vi "Basic_smooth.vi"(0 "Smoothing":enum16{"Linear", "Logarithmic"}(ring), 2 "X array in":dbl[](array[numeric]) format="%.2f", 3 "Y array in":dbl[](array[numeric]) format="%.2f", 4 "No of estimates output":i32=1) -> (5 "X array Out":dbl[](array[numeric]) format="%.2f", 6 "Y array Out":dbl[](array[numeric]) format="%.2f")   [LabVIEW 2010]
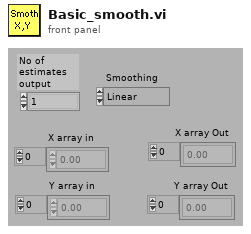
[diagram p1: front panel]
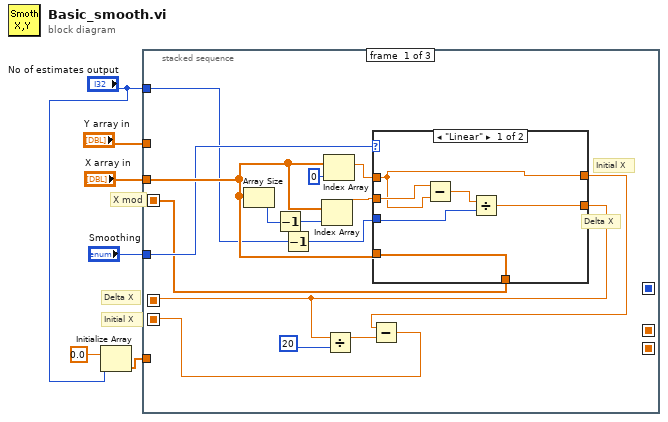
[diagram p0: block diagram]
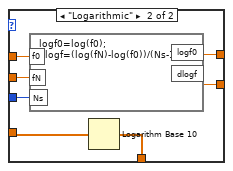
[diagram p2: hidden frame]
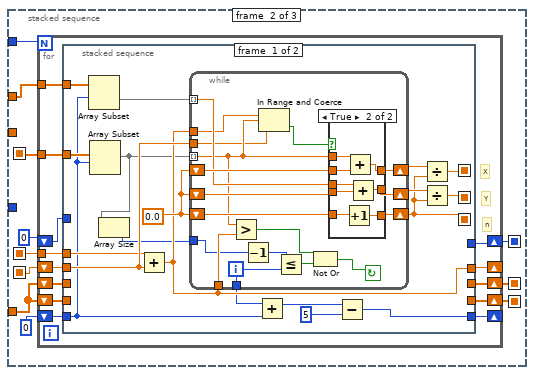
[diagram p3: hidden frame]
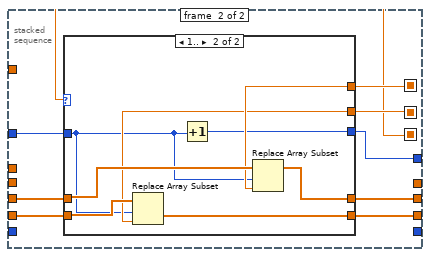
[diagram p5: hidden frame]
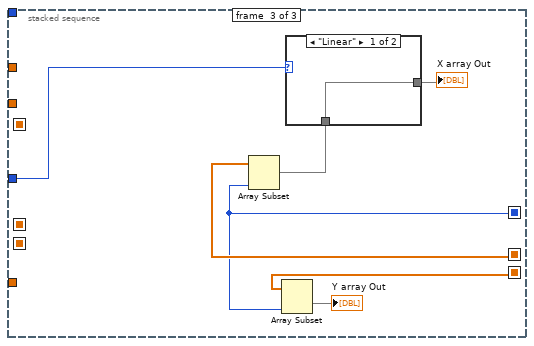
[diagram p7: hidden frame]
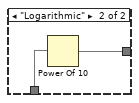
[diagram p8: hidden frame]
diagram:
  # "Initial X"
  # "Delta X"
  # "X mod"
  n1 = Initialize Array(0.0, "No of estimates output") -> (w2:dbl[])
  n2 = stacked-sequence {
    seq-local: [w11 _ _] -> [_ w43 _]
    seq-local: [w7 _ _] -> [_ w42 _]
    seq-local: [w14 _ _] -> [_ w44 _]
    seq-local: [_ w39 _] -> [_ _ w129]
    seq-local: [_ w38 _] -> [_ _ w130]
    seq-local: [_ w35 _] -> [_ _ w128]
    tunnel: "X array in" -> [w16 _ _]
    tunnel: "Smoothing" -> [w15 _ w132]
    tunnel: "No of estimates output" -> [w13 w37 _]
    tunnel: "Y array in" -> [_ w45 _]
    tunnel: w2 -> [_ w41 _]
    frame #0 {
      # "Delta X"
      # "Initial X"
      n3 = Array Size(array=w16) -> (size(s)=w20:i32)
      n4 = Decrement(x=w20) -> (x-1=w19:i32)
      n5 = Decrement(x=w13) -> (x-1=w12:i32)
      n6 = Index Array(array=w16, index=w19) -> (element=w17:dbl)
      n7 = Index Array(array=w16, index=0) -> (element=w18:dbl)
      n8 = case shown="\"Linear\"" w15 {
        tunnel: w18 -> [w23 w34]
        tunnel: w17 -> [w25 w33]
        tunnel: w12 -> [w26 w32]
        tunnel: [w24 w31] -> w11
        tunnel: [w23 w30] -> w8
        tunnel: w16 -> [w22 w29]
        tunnel: [w22 w28] -> w14
        frame "Linear" {
          n9 = Subtract(x=w25, y=w23) -> (x-y=w27:dbl)
          n10 = Divide(x=w27, y=w26) -> (x/y=w24:dbl)
        }
        frame "Logarithmic" {
          n11 = formula code="logf0=log(f0);\ndlogf=(log(fN)-log(f0))/(Ns-1);"("f0"=w34, "fN"=w33, "Ns"=w32) -> ("dlogf"=w31:dbl, "logf0"=w30:dbl)
          n12 = Logarithm Base 10(1:w29) -> (0:w28:dbl[])
        }
      }
      n13 = Divide(x=w11, y=20) -> (x/y=w9:dbl)
      n14 = Subtract(x=w8, y=w9) -> (x-y=w7:dbl)
    }
    frame #1 {
      n15 = for {
        N: w37 -> [_]
        shift-right: [w57] -> _
        shift-left: w42 -> [w58]
        shift-right: [w55] -> w39
        shift-left: w41 -> [w48]
        shift-right: [w54] -> w38
        shift-left: w41 -> [w53]
        tunnel: w43 -> [w56]
        shift-right: [w52] -> _
        shift-left: 0 -> [w51]
        tunnel: w45 -> [w50]
        tunnel: w44 -> [w49]
        shift-right: [w46] -> w35
        shift-left: 0 -> [w47]
        # "n"
        # "Y"
        # "X"
        n16 = stacked-sequence {
          seq-local: [w70 _] -> [_ w111]
          seq-local: [w69 _] -> [_ w110]
          seq-local: [w68 _] -> [_ w107]
          tunnel: w58 -> [w73 _]
          tunnel: [w72 _] -> w57
          tunnel: w56 -> [w71 _]
          tunnel: [_ w115] -> w55
          tunnel: w48 -> [_ w114]
          tunnel: [_ w113] -> w54
          tunnel: w53 -> [_ w112]
          tunnel: [w64 _] -> w52
          tunnel: w51 -> [w61 _]
          tunnel: w50 -> [w63 _]
          tunnel: w49 -> [w62 _]
          tunnel: w47 -> [_ w109]
          tunnel: [_ w108] -> w46
          frame #0 {
            w74 = 0.0
            n17 = Array Subset(array=w63, index=w61) -> (w75:dbl[])  [unwired: 1 in]
            n18 = Array Subset(array=w62, index=w61) -> (w66:dbl[])  [unwired: 1 in]
            n19 = Array Size(array=w66) -> (size(s)=w65:i32)
            n20 = Add(x=w71, y=w73) -> (x+y=w72:dbl)
            n21 = while {
              tunnel: w65 -> [w86]
              tunnel: [w87] -> w60
              tunnel: w72 -> [w88]
              tunnel: w75 -> [w89] mode=indexing
              tunnel: w66 -> [w80] mode=indexing
              tunnel: w72 -> [w81]
              tunnel: w73 -> [w79]
              shift-left: w74 -> [w90]
              shift-right: [w91] -> w76
              shift-left: w74 -> [w95]
              shift-right: [w92] -> w77
              shift-left: w74 -> [w94]
              shift-right: [w93] -> w68
              i -> [w87]
              stop <- w82 continue-if-true
              n22 = Greater?(x=w80, y=w88) -> (0:w84:bool)
              n23 = Decrement(x=w86) -> (x-1=w85:i32)
              n24 = In Range and Coerce(upper limit=w81, x=w80, lower limit=w79) -> (In Range?=w78:bool)  [unwired: 1 out]
              n25 = Less Or Equal?(x=w85, y=w87) -> (x <= y?=w83:bool)
              n26 = Not Or(1:w83, 2:w84) -> (0:w82:bool)
              n27 = case shown="True" w78 {
                tunnel: w94 -> [w97 w103]
                tunnel: [w97 w104] -> w93
                tunnel: [w98 w105] -> w92
                tunnel: w95 -> [w98 w106]
                tunnel: [w96 w100] -> w91
                tunnel: w90 -> [w96 w101]
                tunnel: w80 -> [_ w102]
                tunnel: w89 -> [_ w99]
                frame False {
                }
                frame True {
                  n28 = Increment(x=w103) -> (x+1=w104:dbl)
                  n29 = Add(x=w102, y=w101) -> (x+y=w100:dbl)
                  n30 = Add(x=w99, y=w106) -> (x+y=w105:dbl)
                }
              }
            }
            n31 = Add(x=w60, y=w61) -> (x+y=w59:i32)
            n32 = Subtract(x=w59, y=5) -> (x-y=w64:i32)
            n33 = Divide(x=w76, y=w68) -> (x/y=w70:dbl)
            n34 = Divide(x=w77, y=w68) -> (x/y=w69:dbl)
          }
          frame #1 {
            n35 = case shown="1.." w107 {
              tunnel: [w118 w126] -> w115
              tunnel: w114 -> [w118 w125]
              tunnel: [w117 w121] -> w113
              tunnel: w112 -> [w117 w122]
              tunnel: w111 -> [_ w124]
              tunnel: w110 -> [_ w120]
              tunnel: w109 -> [w116 w119]
              tunnel: [w116 w123] -> w108
              frame ..0 {
              }
              frame 1.. {
                n36 = Replace Array Subset(array=w122, new element=w120, index=w119) -> (w121:dbl[])
                n37 = Increment(x=w119) -> (x+1=w123:i32)
                n38 = Replace Array Subset(array=w125, new element=w124, index=w119) -> (w126:dbl[])
              }
            }
          }
        }
      }
    }
    frame #2 {
      n39 = Array Subset(array=w129, length=w128) -> (w127:dbl[])  [unwired: 1 in]
      n40 = Array Subset(array=w130, length=w128) -> (→"Y array Out":dbl[])  [unwired: 1 in]
      n41 = case shown="\"Linear\"" w132 {
        tunnel: w127 -> [w134 w136]
        tunnel: [w134 w135] -> w133
        frame "Linear" {
        }
        frame "Logarithmic" {
          n42 = Power Of 10(x=w136) -> (10^x=w135:dbl[])
        }
      }
      "X array Out" <- w133
    }
  }
